vi "PH_BeamlineController.PC Accept.vi"(0 "i ref in":refnum<vi>, 5 "error in (no error)":errorcluster) -> (14 "i ref out":refnum<vi>, 19 "error out":errorcluster)   [LabVIEW 2014, in "PH_BeamlineController.lvlib"]
doc: "This VI writes incoming Information to own Attributes if the new value differs from the stored."
uses:
  PH_BeamlineController.lvlib
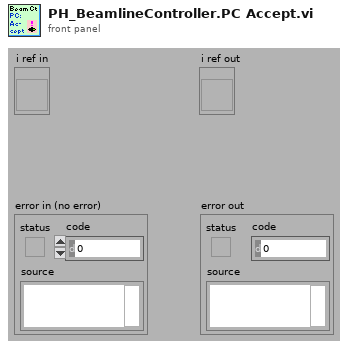
[diagram p1: front panel]
types:
  T1 = typedef "PH_BeamlineController.lvlib/PH_BeamlineController.i attribute.ctl" = cluster{"Vacuum Exp LB":cluster{"Channel":string, "Limit [mbar]":dbl, "Pressure [mbar]":dbl, "GUI Ref":refnum<vi>}, "Sources":T2[], "PA DP Targets":T4[], "Path":cluster{"Source":T3, "PA DP Target":T5, "Target":T6}, "Targets":cluster{"Name":T6, "GUI Ref":refnum<vi>, "Current State":bool, "Wanted State":bool, "Enabled":bool}[], "Status Tags":cluster{"Name":string, "Status":T7}[], "special GUI Refs":T8}
  T2 = typedef "PH_BeamlineController.lvlib/PH_BeamlineController.Source Attributes.ctl" = cluster{"Name":T3, "GUI Ref":refnum<vi>, "Current State":bool, "Wanted State":bool}
  T3 = typedef "PH_BeamlineController.lvlib/PH_BeamlineController.Sources.ctl" = enum16{"None", "YLF", "fs-Frontend", "ns-Frontend", "YLF and ns-Frontend", "fs- and ns-Frontend"}
  T4 = typedef "PH_BeamlineController.lvlib/PH_BeamlineController.PA DP Target Attributes.ctl" = cluster{"Name":T5, "GUI Ref":refnum<vi>, "Current State":bool, "Wanted State":bool, "Enabled":bool}
  T5 = typedef "PH_BeamlineController.lvlib/PH_BeamlineController.PA DP Targets.ctl" = enum16{"None", "Dump PA Delayed Beam", "Dump PA Undelayed Beam", "Dumps PA Delayed and Undelayed Beam"}
  T6 = typedef "PH_BeamlineController.lvlib/PH_BeamlineController.Targets.ctl" = enum16{"None", "PreAmp", "Dump Exp Laserlab", "Exp Laserlab", "Calorimeter", "Dump Exp Laserbay", "Exp Laserbay", "Dump Exp Z6", "Exp Z6"}
  T7 = typedef "PH_StatusHandler.lvlib/PH_StatusHandler.Status.ctl" = i16
  T8 = typedef "PH_BeamlineController.lvlib/PH_BeamlineController.special GUI Refs.ctl" = cluster{"PA-Backreflection-Meas":refnum<vi>, "fs_Synchrolock_Watch":refnum<vi>}
  T9 = cluster{"Name":T6, "GUI Ref":refnum<vi>, "Current State":bool, "Wanted State":bool, "Enabled":bool}[]
  T10 = cluster{"Name":T6, "GUI Ref":refnum<vi>, "Current State":bool, "Wanted State":bool, "Enabled":bool}
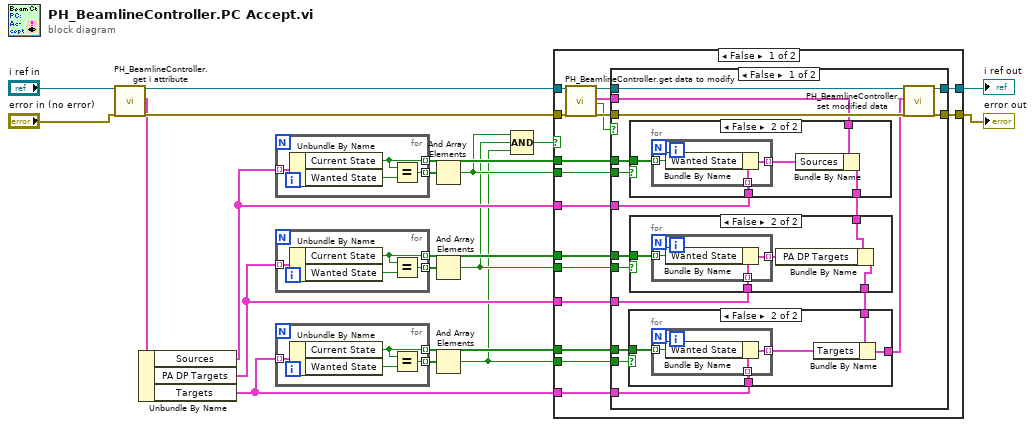
[diagram p0: block diagram]
diagram:
  n1 = call "PH_BeamlineController.get i attribute.vi"("i ref in"="i ref in", "error in (no error)"="error in (no error)") -> ("i ref out"=w14:refnum<vi>, "i attribute"=w17:T1, "error out"=w18:errorcluster)  [unwired: 15 in]
  n2 = Unbundle By Name(w17) -> ("Sources"=w12:T2[], "PA DP Targets"=w5:T4[], "Targets"=w6:T9)
  n3 = for {
    tunnel: w12 -> [w24] mode=indexing
    tunnel: [w22] -> w16 mode=indexing
    tunnel: [w21] -> w11 mode=indexing
    n4 = Unbundle By Name(w24) -> ("Current State"=w21:bool, "Wanted State"=w23:bool)
    n5 = Equal?(x=w21, y=w23) -> (x = y?=w22:bool)
  }
  n6 = for {
    tunnel: w5 -> [w28] mode=indexing
    tunnel: [w26] -> w10 mode=indexing
    tunnel: [w25] -> w8 mode=indexing
    n7 = Unbundle By Name(w28) -> ("Current State"=w25:bool, "Wanted State"=w27:bool)
    n8 = Equal?(x=w25, y=w27) -> (x = y?=w26:bool)
  }
  n9 = for {
    tunnel: w6 -> [w32] mode=indexing
    tunnel: [w30] -> w9 mode=indexing
    tunnel: [w29] -> w7 mode=indexing
    n10 = Unbundle By Name(w32) -> ("Current State"=w29:bool, "Wanted State"=w31:bool)
    n11 = Equal?(x=w29, y=w31) -> (x = y?=w30:bool)
  }
  n12 = And Array Elements(Boolean array=w16) -> (logical AND=w4:bool)
  n13 = And Array Elements(Boolean array=w10) -> (logical AND=w3:bool)
  n14 = And Array Elements(Boolean array=w9) -> (logical AND=w2:bool)
  n15 = Compound Arithmetic op=AND(w4, w3, w2) -> (w1:bool)
  n16 = case shown="False" w1 {
    tunnel: w18 -> [w49 w96]
    tunnel: [w48 w96] -> w15
    tunnel: w14 -> [w46 w97]
    tunnel: [w44 w97] -> w13
    tunnel: w12 -> [w41 _]
    tunnel: w11 -> [w40 _]
    tunnel: w4 -> [w39 _]
    tunnel: w8 -> [w38 _]
    tunnel: w3 -> [w37 _]
    tunnel: w2 -> [w36 _]
    tunnel: w7 -> [w35 _]
    tunnel: w6 -> [w34 _]
    tunnel: w5 -> [w33 _]
    frame False {
      n17 = call "PH_BeamlineController.get data to modify.vi"("i ref in"=w46, "error in (no error)"=w49) -> ("i ref out"=w45:refnum<vi>, "i attribute"=w42:T1, "timed out"=w43:bool, "error out"=w47:errorcluster)  [unwired: 14 in]
      n18 = case shown="False" w43 {
        tunnel: [w66 w94] -> w48
        tunnel: w47 -> [w65 w94]
        tunnel: w45 -> [w64 w95]
        tunnel: [w63 w95] -> w44
        tunnel: w42 -> [w62 _]
        tunnel: w41 -> [w61 _]
        tunnel: w40 -> [w60 _]
        tunnel: w39 -> [w59 _]
        tunnel: w38 -> [w58 _]
        tunnel: w37 -> [w57 _]
        tunnel: w36 -> [w51 _]
        tunnel: w35 -> [w52 _]
        tunnel: w34 -> [w53 _]
        tunnel: w33 -> [w55 _]
        frame False {
          n19 = case shown="False" w59 {
            tunnel: w62 -> [w85 w90]
            tunnel: [w85 w89] -> w56
            tunnel: w61 -> [_ w88]
            tunnel: w60 -> [_ w86]
            frame True {
            }
            frame False {
              n20 = for {
                tunnel: w88 -> [w93] mode=indexing
                tunnel: [w92] -> w87 mode=indexing
                tunnel: w86 -> [w91] mode=indexing
                n21 = Bundle By Name(cluster=w93, "Wanted State"=w91) -> (w92:T2)
              }
              n22 = Bundle By Name(cluster=w90, "Sources"=w87) -> (w89:T1)
            }
          }
          n23 = case shown="False" w57 {
            tunnel: w56 -> [w76 w81]
            tunnel: [w76 w80] -> w54
            tunnel: w55 -> [_ w79]
            tunnel: w58 -> [_ w77]
            frame True {
            }
            frame False {
              n24 = for {
                tunnel: w79 -> [w84] mode=indexing
                tunnel: [w83] -> w78 mode=indexing
                tunnel: w77 -> [w82] mode=indexing
                n25 = Bundle By Name(cluster=w84, "Wanted State"=w82) -> (w83:T4)
              }
              n26 = Bundle By Name(cluster=w81, "PA DP Targets"=w78) -> (w80:T1)
            }
          }
          n27 = case shown="False" w51 {
            tunnel: w54 -> [w67 w72]
            tunnel: [w67 w71] -> w50
            tunnel: w53 -> [_ w70]
            tunnel: w52 -> [_ w68]
            frame True {
            }
            frame False {
              n28 = for {
                tunnel: w70 -> [w75] mode=indexing
                tunnel: [w74] -> w69 mode=indexing
                tunnel: w68 -> [w73] mode=indexing
                n29 = Bundle By Name(cluster=w75, "Wanted State"=w73) -> (w74:T10)
              }
              n30 = Bundle By Name(cluster=w72, "Targets"=w69) -> (w71:T1)
            }
          }
          n31 = call "PH_BeamlineController.set modified data.vi"("i ref in"=w64, "i attribute"=w50, "error in (no error)"=w65) -> ("i ref out"=w63:refnum<vi>, "error out"=w66:errorcluster)  [unwired: 15 in]
        }
        frame True {
        }
      }
    }
    frame True {
    }
  }
  "error out" <- w15
  "i ref out" <- w13
